vi "Write Model case running.vi"(7 "Send any changes now? (F)":bool, 8 "error in (no error)":errorcluster, 10 "Model case running":string, 11 "Fiber Auto Collimation state data in":refnum<class "Fiber Auto Collimation state data.lvclass">) -> (0 "error out":errorcluster, 3 "Fiber Auto Collimation state data out":refnum<class "Fiber Auto Collimation state data.lvclass">)   [LabVIEW 2018, in "Fiber Auto Collimation state data.lvclass"]
doc: "This is the current state running on the main Model loop. If nothing is running, then this should be set to \"Idle\"."
uses:
  Fiber Auto Collimation state data.lvclass
  Fiber Auto Collimation state data.lvclass/Fiber Auto Collimation state data.ctl
  Tracked state data.ctl
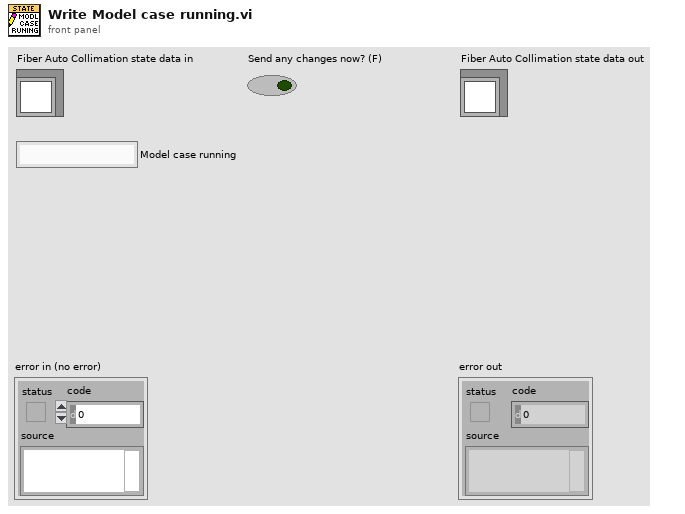
[diagram p1: front panel]
types:
  T1 = typedef "Fiber Auto Collimation state data.lvclass/Tracked state data.ctl" = enum16{"No update", "Permission level", "Username", "Test running", "DUT Serial", "Test status", "MOM Lot", "Loaded test recipe", "Model case running", "Station status", "BV data", "Defect Identify data", "Axis Position data", "Fiber Ass PN", "Operator", "RunTime", "VBAI", "Steps Cycle Time"}
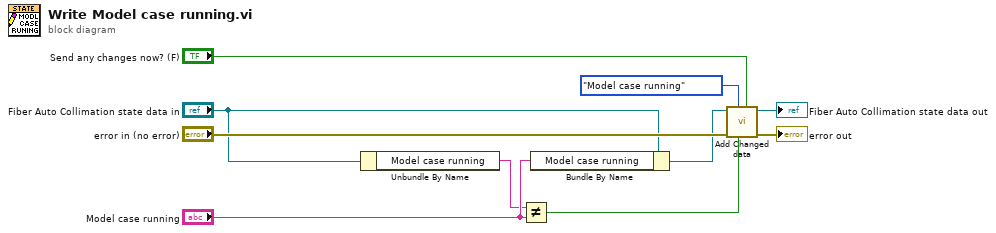
[diagram p0: block diagram]
diagram:
  n1 = Unbundle By Name("Fiber Auto Collimation state data in") -> ("Model case running"=w2:string)
  n2 = Not Equal?(x=w2, y="Model case running") -> (x != y?=w3:bool)
  n3 = Bundle By Name(cluster="Fiber Auto Collimation state data in", "Model case running"="Model case running") -> (w6:refnum<class "Fiber Auto Collimation state data.lvclass">)
  n4 = call "Add Changed data.vi"("Send any changes now? (F)"="Send any changes now? (F)", "Data changed?"=w3, "Data type"=Tracked_state_data."Model case running", "error in (no error)"="error in (no error)", "Fiber Auto Collimation state data in"=w6) -> ("error out"=→"error out":errorcluster, "Fiber Auto Collimation state data out"=→"Fiber Auto Collimation state data out":refnum<class "Fiber Auto Collimation state data.lvclass">)  [unwired: 5 in]
